vi "Write Receive Binary Data queue.vi"(8 "error in (no error)":errorcluster, 10 "Receive Binary Data":refnum<queue>, 11 "WebSocket Data Model in":refnum<class "WebSocket Data Model.lvclass">) -> (0 "error out":errorcluster, 3 "WebSocket Data Model out":refnum<class "WebSocket Data Model.lvclass">)   [LabVIEW 2021, in "WebSockets.lvlib" / "WebSocket Data Model.lvclass"]
uses:
  WebSocket Data Model.lvclass
  WebSocket Data Model.lvclass/WebSocket Data Model.ctl
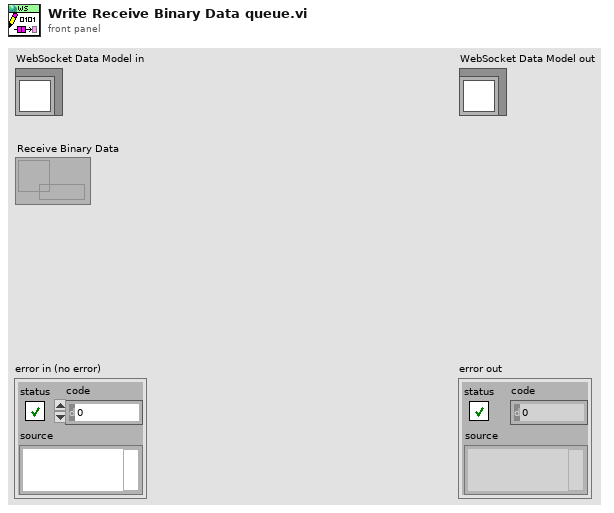
[diagram p1: front panel]
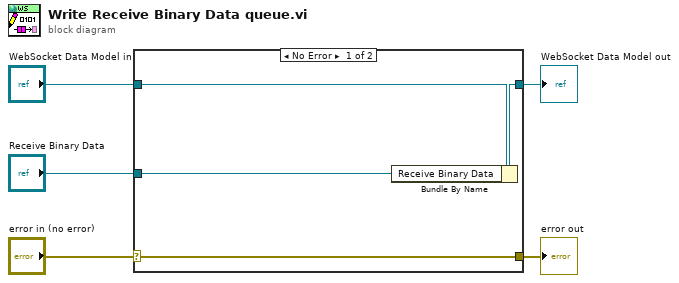
[diagram p0: block diagram]
diagram:
  n1 = case shown="No Error" "error in (no error)" {
    selector: "error in (no error)" -> [w9 w10]
    tunnel: [w9 w10] -> w4
    tunnel: [w7 w11] -> w2
    tunnel: "WebSocket Data Model in" -> [w8 w11]
    tunnel: "Receive Binary Data" -> [w6 _]
    frame No Error {
      n2 = Bundle By Name(cluster=w8, "Receive Binary Data"=w6) -> (w7:refnum<class "WebSocket Data Model.lvclass">)
    }
    frame Error {
    }
  }
  "error out" <- w4
  "WebSocket Data Model out" <- w2
